vi "Test Suite Disable Method of Suite From Project.vi"(8 "error in (no error)":errorcluster, 11 "Test Case In":refnum<class "LUnit Test Suite Tests.lvclass">) -> (0 "error out":errorcluster, 3 "Test Case Out":refnum<class "LUnit Test Suite Tests.lvclass">)   [LabVIEW 2020, in "LUnit Test Suite Tests.lvclass"]
uses:
  LUnit Test Suite Tests.lvclass
  C:/Program Files (x86)/National Instruments/LabVIEW 2020/vi.lib/Astemes/LUnit/Test Case.lvclass
  <vilib>/Astemes/LUnit/Test Case.lvclass/Test Case.ctl
  <vilib>/Astemes/LUnit/Palette/Fail.vi
  <vilib>/Astemes/LUnit/Palette/Pass.vi
  <vilib>/Astemes/LUnit/Set Assertion Type.vi
  <vilib>/Astemes/LUnit/Add test result.vi
  <vilib>/Astemes/LUnit/LUnit Record Assertion Result.vi
  <vilib>/Astemes/LUnit/LUnit Aggregate Assertion Results.vi
  <vilib>/Astemes/LUnit/Method Result/LUnit Merge Status.vi
  <vilib>/Astemes/LUnit/LUnit Concatenate result strings.vi
  Mock Result Observer/Mock Result Observer.lvclass
  C:/git/astemes-lunit/source/Core/Result Observer/Result Observer.lvclass
  Core/LUnit Test Suite/LUnit Test Suite.lvclass
  <vilib>/Astemes/LUnit/Test Case.lvclass
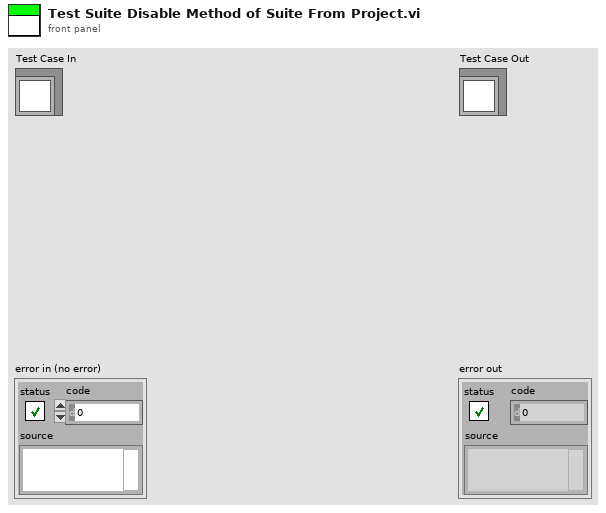
[diagram p1: front panel]
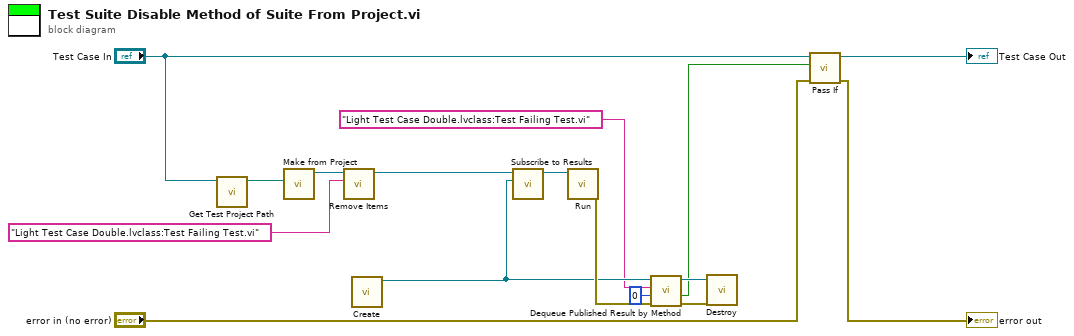
[diagram p0: block diagram]
diagram:
  n1 = call "Get Test Project Path.vi"("LUnit Test Suite Tests in"="Test Case In") -> ("appended path"=w10:path)  [unwired: 10 in]
  n2 = call "Make from Project.vi"("Project Path"=w10) -> ("LUnit Test Suite Out"=w13:refnum<class "LUnit Test Suite.lvclass">)  [unwired: 9 in, 1 out]
  n3 = call "Remove Items.vi"("Methods"="Light Test Case Double.lvclass:Test Failing Test.vi", "LUnit Test Suite In"=w13) -> ("LUnit Test Suite Out"=w8:refnum<class "LUnit Test Suite.lvclass">)  [unwired: 8 in, 1 out]
  n4 = call "Create.vi"() -> ("Mock Result Observer out"=w6:refnum<class "Mock Result Observer.lvclass">)  [unwired: 10 in, 1 out]
  n5 = call-dynamic "Subscribe to Results.vi"("Result Observer"=w6, "LUnit Test Suite In"=w8) -> ("LUnit Test Suite Out"=w9:refnum<class "LUnit Test Suite.lvclass">)  [unwired: 8 in, 1 out]
  n6 = call-dynamic "Run.vi"("LUnit Test Suite In"=w9) -> ("error out"=w7:errorcluster)  [unwired: 9 in, 1 out]
  n7 = call "Dequeue Published Result by Method.vi"("error in (no error)"=w7, "timeout in ms"=0, "Method Name"="Light Test Case Double.lvclass:Test Failing Test.vi", "Mock Result Observer In"=w6) -> ("error out"=w4:errorcluster, "timed out?"=w3:bool, "Mock Result Observer Out"=w5:refnum<class "Mock Result Observer.lvclass">)  [unwired: 4 in, 1 out]
  n8 = call "Destroy.vi"("error in (no error)"=w4, "Mock Result Observer in"=w5) -> ()  [unwired: 8 in, 2 out]
  n9 = call <vilib>:"Pass If.vi"("error in (no error)"="error in (no error)", "Pass?"=w3, "LUnit Test Case In"="Test Case In") -> ("error out"=→"error out":errorcluster, "LUnit Test Case Out"=→"Test Case Out":refnum<class "LUnit Test Suite Tests.lvclass">)  [unwired: 7 in]
